vi "SFC_Process Update Command.vi"(0 "Traceability 引用句柄":refnum<k24>, 1 "Type":string, 2 "UserNo":string, 5 "IntSerialNo":string, 7 "ProdOrder":string, 9 "Process":string, 11 "error in (no error)":errorcluster caption="错误输入（无错误）", 12 "AssemblyNo":string) -> (4 "Traceability 引用句柄输出":refnum<k24>, 6 "SFC_ProcessUpdateCommand":string, 15 "error out":errorcluster caption="错误输出")   [LabVIEW 2014, in "Traceability.lvlib"]
uses:
  D:/webservice/Traceability.dll
  Traceability.dll
  Traceability.lvlib
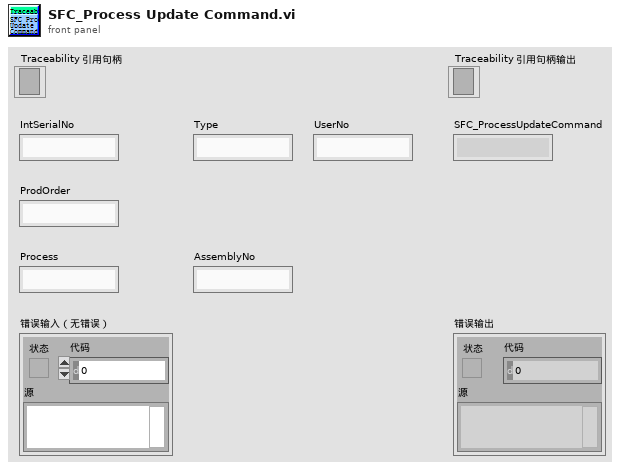
[diagram p1: front panel]
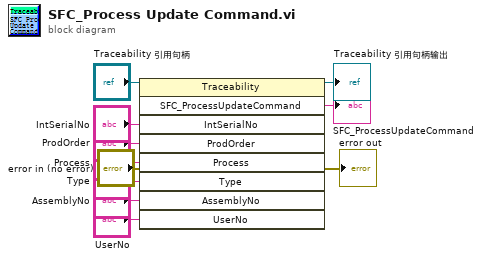
[diagram p0: block diagram]
diagram:
  n1 = invoke class="Traceability" method="SFC_ProcessUpdateCommand"(reference="Traceability 引用句柄", error in="error in (no error)", "IntSerialNo"="IntSerialNo", "ProdOrder"="ProdOrder", "Process"="Process", "Type"="Type", "AssemblyNo"="AssemblyNo", "UserNo"="UserNo") -> (reference out=→"Traceability 引用句柄输出":refnum<k24>, error out=→"error out":errorcluster, "SFC_ProcessUpdateCommand"=→"SFC_ProcessUpdateCommand":string)  [unwired: 1 in, 6 out]
